vi "Create Measurement Services.vi"(8 "error in (no error)":errorcluster, 10 "Measurement Service Version":string[](array[string]), 11 "gRPC ID in":T1) -> (0 "error out":errorcluster, 2 "IMeasurementService Array out":refnum<class "IMeasurementService.lvclass">[](array[class]), 3 "gRPC ID out":T1)   [LabVIEW 2020, in "MeasurementLink Measurement Server.lvlib"]
uses:
  MeasurementLink Measurement Server.lvlib
  Classes/IMeasurementService/IMeasurementService.lvclass
  <vilib>/gRPC/LabVIEW gRPC Library/Shared/grpcId.ctl
  Classes/MeasurementServiceV2/MeasurementServiceV2.lvclass
  Classes/MeasurementServiceV1/MeasurementServiceV1.lvclass
  <vilib>/gRPC/LabVIEW gRPC Library/grpc-lvsupport-release.lvlib
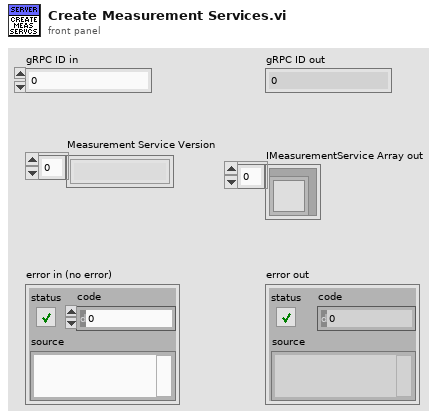
[diagram p1: front panel]
types:
  T1 = typedef "grpc-lvsupport-release.lvlib/grpcId.ctl" = u64
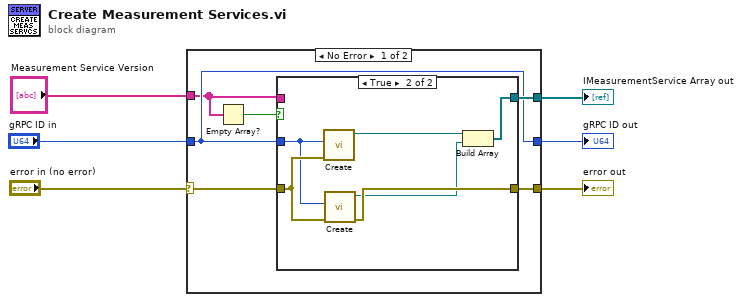
[diagram p0: block diagram]
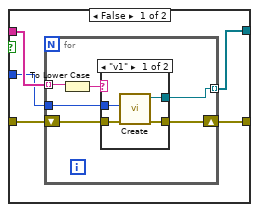
[diagram p2: hidden frame]
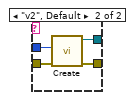
[diagram p3: hidden frame]
diagram:
  n1 = case shown="No Error" "error in (no error)" {
    selector: "error in (no error)" -> [w11 w39]
    tunnel: [w12 w39] -> w5
    tunnel: [w10 _] -> w4
    tunnel: "gRPC ID in" -> [w9 w38]
    tunnel: [w9 w38] -> w2
    tunnel: "Measurement Service Version" -> [w7 _]
    frame No Error {
      n2 = Empty Array?(array=w7) -> (empty?=w8:bool)
      n3 = case shown="True" w8 {
        tunnel: [w14 w37] -> w12
        tunnel: w11 -> [w15 w36]
        tunnel: [w13 w33] -> w10
        tunnel: w9 -> [w16 w32]
        tunnel: w7 -> [w17 _]
        frame False {
          n4 = for {
            tunnel: w17 -> [w23] mode=indexing
            tunnel: w16 -> [w21]
            tunnel: [w18] -> w13 mode=indexing
            shift-right: [w19] -> w14
            shift-left: w15 -> [w20]
            n5 = To Lower Case(string=w23) -> (all lower case string=w22:string)
            n6 = case shown="\"v1\"" w22 {
              tunnel: w21 -> [w26 w28]
              tunnel: w20 -> [w27 w31]
              tunnel: [w25 w30] -> w19
              tunnel: [w24 w29] -> w18
              frame "v1" {
                n7 = call "Create.vi"("error in (no error)"=w27, "gRPC ID in"=w26) -> ("error out"=w25:errorcluster, "IMeasurementService out"=w24:refnum<class "IMeasurementService.lvclass">)  [unwired: 7 in, 1 out]
              }
              frame "v2", Default {
                n8 = call "Create.vi"("error in (no error)"=w31, "gRPC ID in"=w28) -> ("error out"=w30:errorcluster, "IMeasurementService out"=w29:refnum<class "IMeasurementService.lvclass">)  [unwired: 7 in, 1 out]
              }
            }
          }
        }
        frame True {
          n9 = call "Create.vi"("error in (no error)"=w36, "gRPC ID in"=w32) -> ("IMeasurementService out"=w35:refnum<class "IMeasurementService.lvclass">)  [unwired: 7 in, 2 out]
          n10 = call "Create.vi"("error in (no error)"=w36, "gRPC ID in"=w32) -> ("error out"=w37:errorcluster, "IMeasurementService out"=w34:refnum<class "IMeasurementService.lvclass">)  [unwired: 7 in, 1 out]
          n11 = Build Array(w35, w34) -> (w33:refnum<class "IMeasurementService.lvclass">[])
        }
      }
    }
    frame Error {
    }
  }
  "error out" <- w5
  "IMeasurementService Array out" <- w4
  "gRPC ID out" <- w2
